vi "Get Full Scale.vi"(8 "error in (no error)":errorcluster, 11 "VISA resource name":refnum<visa-resource-name>) -> (0 "error out":errorcluster, 2 "Full Scale":dbl, 3 "VISA resource name out":refnum<visa-resource-name>)   [LabVIEW 2018, in "MFC Actor.lvlib" / "MFC.lvclass"]
uses:
  MFC.lvclass
  <instrlib>/Sierra Instruments Smart-Trak 100 Series/Sierra Instruments Smart-Trak 100 Series.lvlib
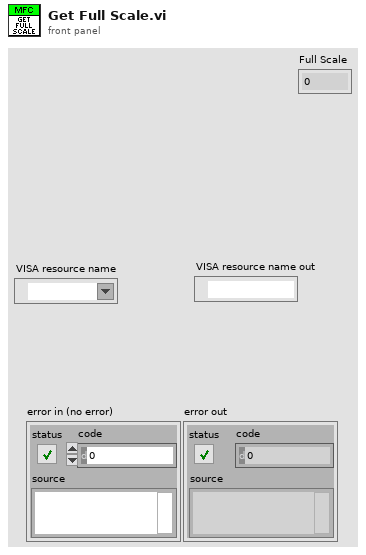
[diagram p1: front panel]
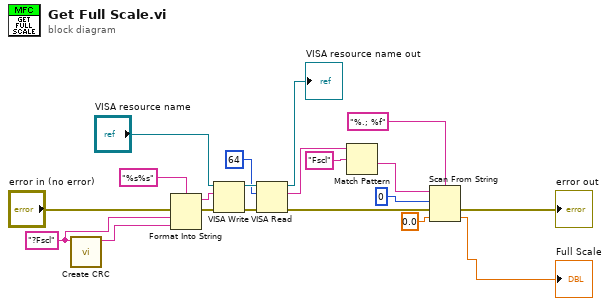
[diagram p0: block diagram]
diagram:
  w18 = "?Fscl" ("multi-line string")
  n1 = call <instrlib>:"Create CRC.vi"("Command String"=w18) -> ("CRC Value"=w14:string)  [unwired: 9 in, 1 out]
  n2 = Format Into String(format string="%s%s", error in="error in (no error)", w18, w14) -> (resulting string=w15:string, error out=w17:errorcluster)  [unwired: 1 in]
  n3 = VISA Write(VISA resource name="VISA resource name", write buffer=w15, error in (no error)=w17) -> (VISA resource name out=w20:refnum<visa-resource-name>, error out=w5:errorcluster)  [unwired: 1 out]
  n4 = VISA Read(VISA resource name=w20, byte count=u32 64, error in (no error)=w5) -> (VISA resource name out=→"VISA resource name out":refnum<visa-resource-name>, read buffer=w13:string, error out=w3:errorcluster)  [unwired: 1 out]
  n5 = Match Pattern(string=w13, regular expression="Fscl") -> (after substring=w12:string)  [unwired: 1 in, 3 out]
  n6 = Scan From String(format string="%.; %f", input string=w12, initial scan location=u32 0, error in=w3, default 1=0.0 ("default value 1")) -> (error out=→"error out":errorcluster, output 1=→"Full Scale":dbl)  [unwired: 2 out]
